vi "SyncTag_2.0 Test.vi"() -> ()   [LabVIEW 2017]
uses:
  <vilib>/Utility/error.llb/DialogType.ctl
  <vilib>/DAQmx/write.llb/DAQmx Write (Digital Wfm 1Chan NSamp).vi
  <vilib>/Waveform/DWDTOps.llb/DWDT Digital Size.vi
  <vilib>/DAQmx/create/channels.llb/DAQmx Create Channel (CO-Pulse Generation-Time).vi
  <vilib>/DAQmx/configure/timing.llb/DAQmx Timing (Implicit).vi
  <vilib>/DAQmx/create/channels.llb/DAQmx Create Channel (DO-Digital Output).vi
  <vilib>/DAQmx/configure/timing.llb/DAQmx Timing (Sample Clock).vi
  <vilib>/Waveform/DWDTOps.llb/DWDT Boolean Array to Digital.vi
  <vilib>/Waveform/DWDTOps.llb/DWDT Uncompress Digital.vi
  <vilib>/DAQmx/miscellaneous.llb/DAQmx Fill In Error Info.vi
panel:
  out "error out 8":errorcluster
  out "error out 7":errorcluster
  out "Numeric":i32
  out "error out 6":errorcluster
  out "error out 5":errorcluster
  out "error out 4":errorcluster
  out "error out 3":errorcluster
  out "error out 2":errorcluster
  out "error out":errorcluster
  in  "Sync Tagging":T1(tab)
  out "Minimum tagging period (pws)":u32=87
  out "Total tag data length (pws)":u32=86
  in  "TaggingPeriod (pws)":u32=155
  out "Tag data does NOT fit in period!!!":bool
  in  "Calculate recommended tag settings":bool
  in  "Validate tag settings":bool
  in  "TagMarkerDuration (pws)":i32=10
  in  "stop":bool
  out "Digital Waveform Graph":digitalwaveform(graph)
  in  "Minimum extra tag separation (pws)":u32=1
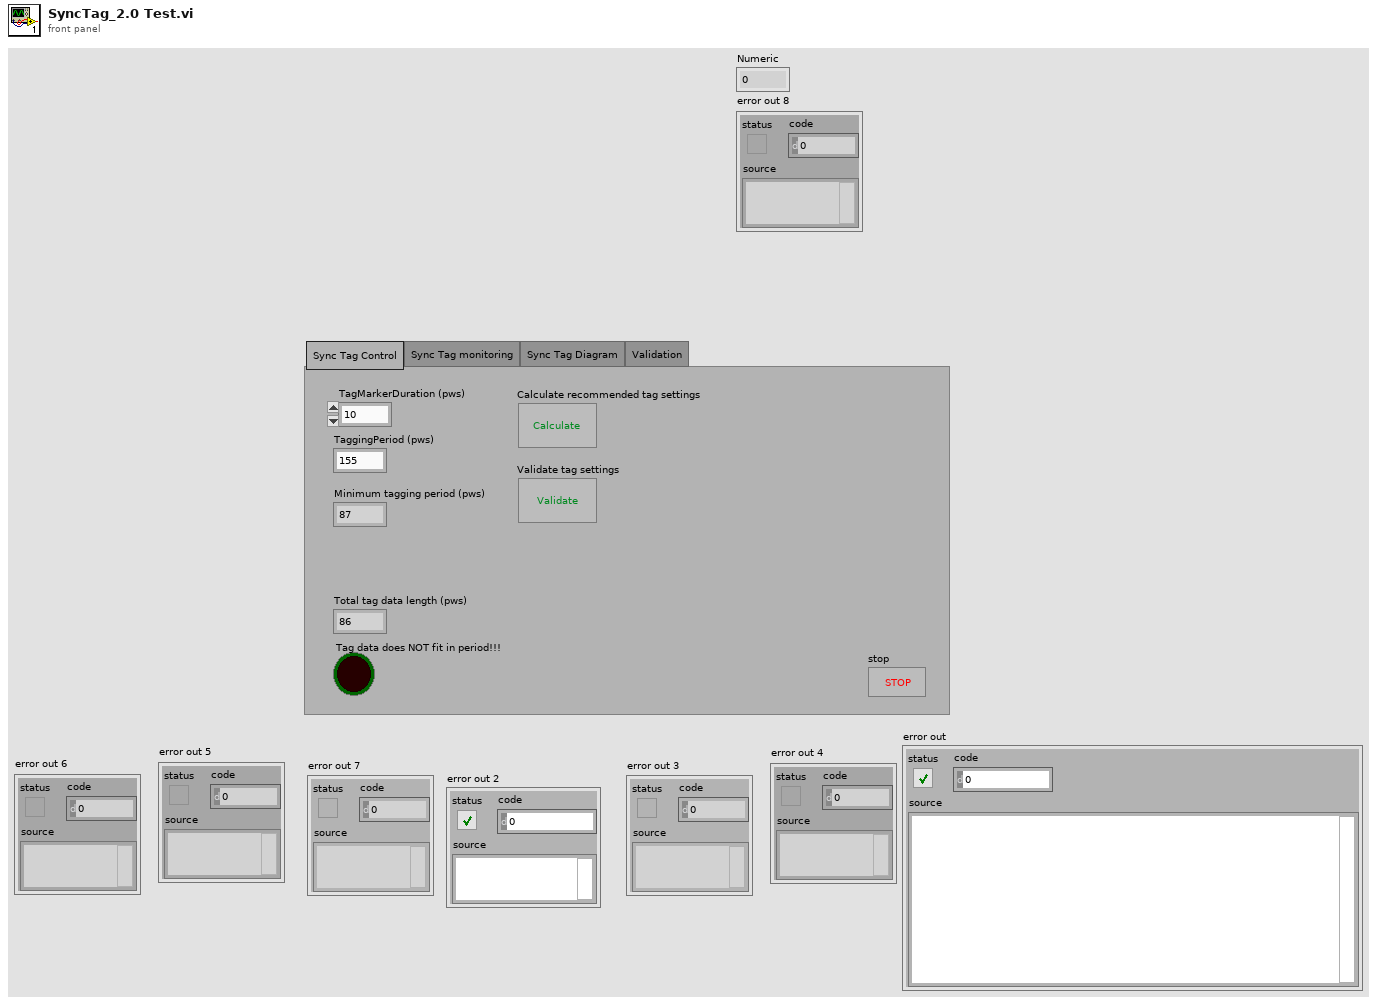
[diagram p1: front panel]
types:
  T1 = enum32{"Sync Tag Control", "Sync Tag monitoring", "Sync Tag Diagram", "Validation"}
  T2 = typedef "DialogType.ctl" = u16
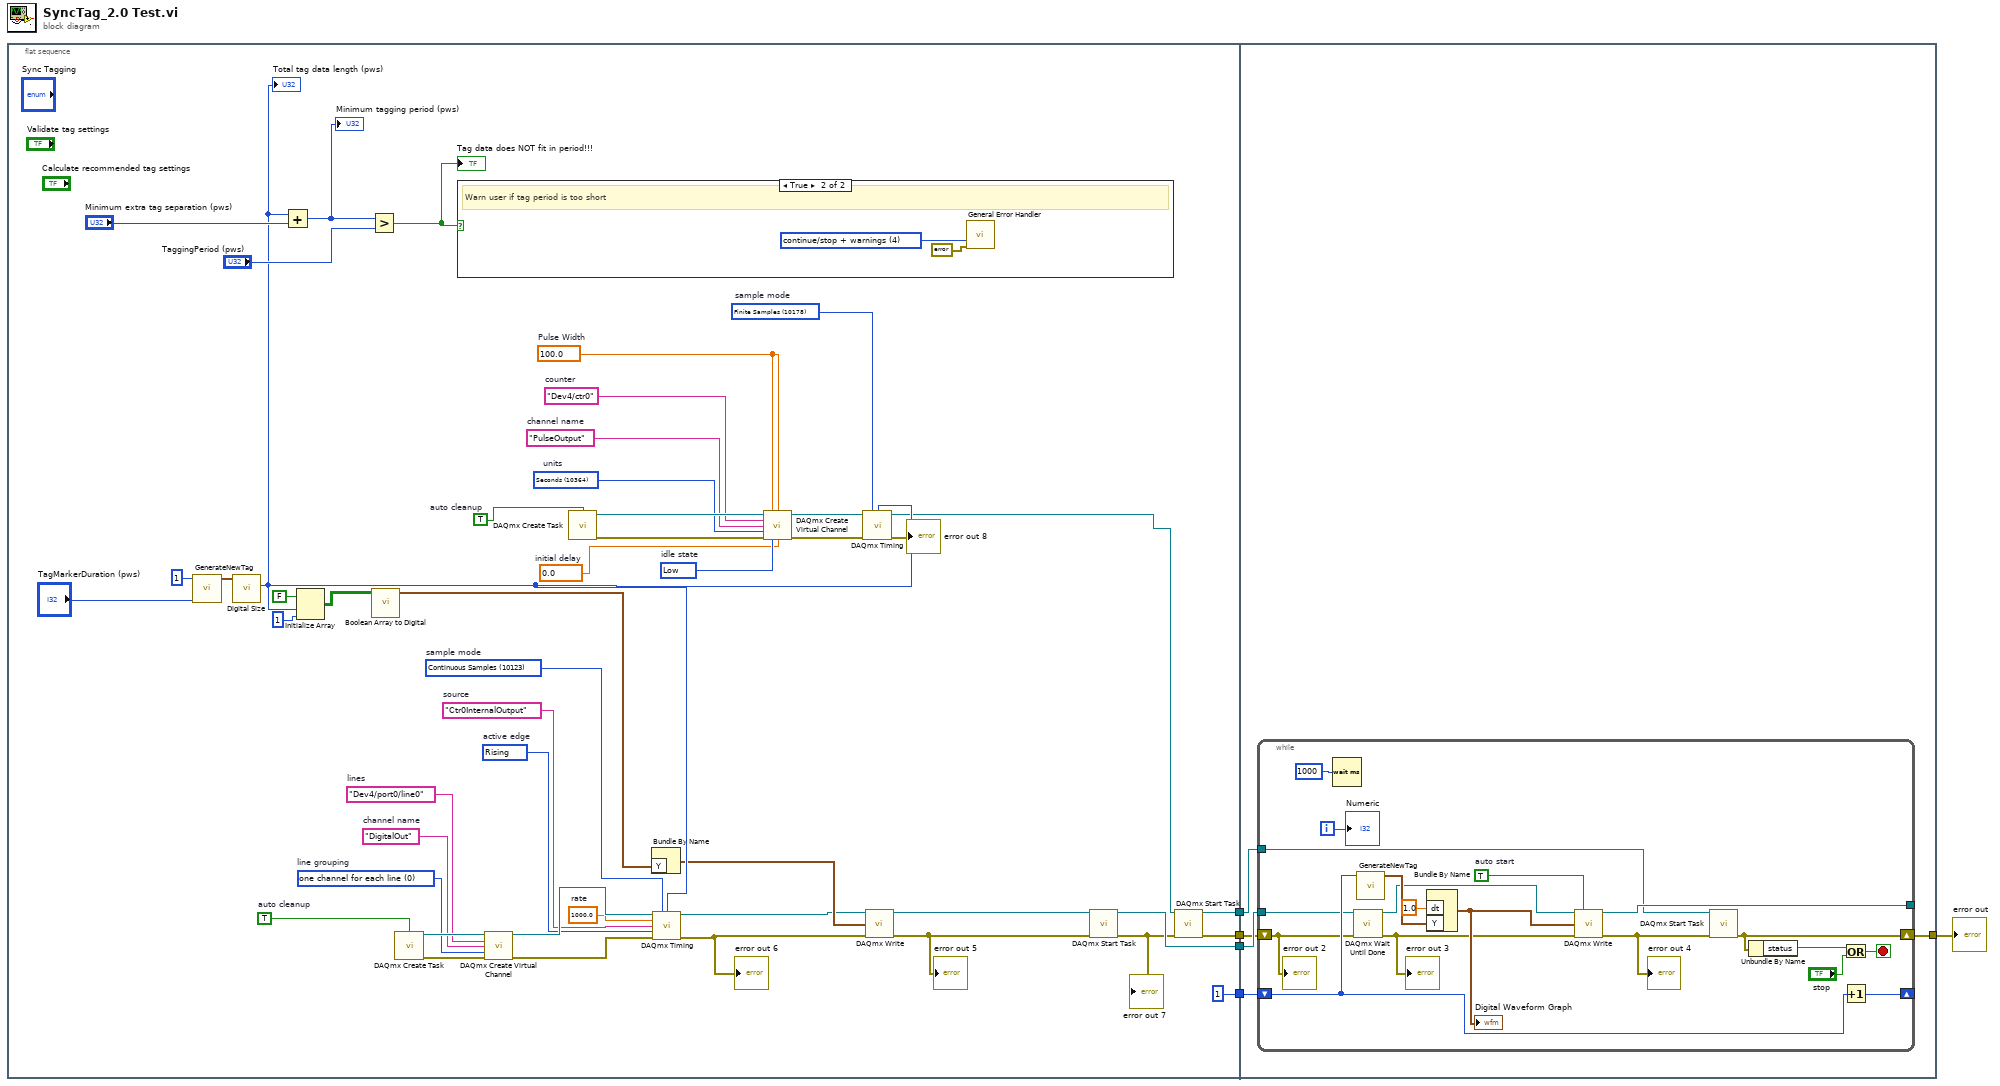
[diagram p0: block diagram]
diagram:
  n1 = flat-sequence {
    tunnel: [w8] -> w5
    tunnel: [u32 1 ("Tag num")] -> w4
    tunnel: [w13] -> w3
    tunnel: [w9] -> w1
    tunnel: w5 -> [w60]
    tunnel: w4 -> [w59]
    tunnel: w3 -> [w58]
    tunnel: [w57] -> w2
    tunnel: w1 -> [w56]
    frame #0 {
      w30 = 10123 items=["Finite Samples"=10178, "Continuous Samples"=10123, "Hardware Timed Single Point"=12522]  # sample mode
      w29 = 1000.0  # rate
      w27 = 10280 items=["Rising"=10280, "Falling"=10171]  # active edge
      w28 = "Ctr0InternalOutput"  # source
      w24 = 0 items=["one channel for each line", "one channel for all lines"]  # line grouping
      w25 = "DigitalOut"  # channel name
      w26 = "Dev4/port0/line0"  # lines
      w23 = TRUE  # auto cleanup
      w22 = 10178 items=["Finite Samples"=10178, "Continuous Samples"=10123, "Hardware Timed Single Point"=12522]  # sample mode
      w21 = 100.0  # Pulse Width
      w16 = 0.0  # initial delay
      w17 = 10214 items=["High"=10192, "Low"=10214]  # idle state
      w18 = 10364 items=["Seconds"=10364, "From Custom Scale"=10065]  # units
      w19 = "PulseOutput"  # channel name
      w20 = "Dev4/ctr0"  # counter
      w15 = TRUE  # auto cleanup
      n2 = call "GenerateNewTag.vi"("TagMarkerDuration (pws)"="TagMarkerDuration (pws)", "Tag num"=u32 1) -> ("digital waveform"=w46:digitalwaveform)  [unwired: 9 in]
      n3 = call-poly <vilib>:"Digital Size.vi"("digital waveform in"=w46) -> ("number of samples"=w47:i32)  [unwired: 7 in, 3 out]
      "Total tag data length (pws)" <- w47
      n4 = Add(x=w47, y="Minimum extra tag separation (pws)") -> (x+y=w53:u32)
      "Minimum tagging period (pws)" <- w53
      n5 = Initialize Array(FALSE, w47, 1 ("dimension size")) -> (w43:bool[][])
      n6 = Greater?(x=w53, y="TaggingPeriod (pws)") -> (0:w52:bool)
      "Tag data does NOT fit in period!!!" <- w52
      n7 = call-poly <vilib>:"Boolean Array to Digital.vi"("boolean array"=w43) -> ("digital waveform"=w44:digitalwaveform)  [unwired: 9 in, 1 out]
      n8 = call <vilib>:"DAQmx Create Task.vi"("auto cleanup"=w23) -> ("task out"=w40:refnum<k21>, "error out"=w39:errorcluster)  [unwired: 13 in]
      n9 = case shown="True" w52 {
        frame False {
        }
        frame True {
          w54 = T2 4 items=["no dialog", "OK message", "continue or stop message", "OK message + warnings", "continue/stop + warnings"] ("type of dialog (OK msg:1)")
          # "Warn user if tag period is too short"
          n10 = call <vilib>:"General Error Handler.vi"("type of dialog (OK msg:1)"=w54, "error in (no error)"=errorcluster {"status"=TRUE, "code"=-1967345148, "source"="Warning! Tag data does not fit in period. \nPlease increase tag period and restart VI."}) -> ()  [unwired: 9 in, 5 out]
        }
      }
      n11 = call-poly <vilib>:"DAQmx Create Virtual Channel.vi"("task in"=w40, "lines"=w26, "name to assign"=w25, "line grouping"=w24, "error in"=w39) -> ("task out"=w42:refnum<k21>, "error out"=w41:errorcluster)  [unwired: 9 in]
      n12 = call <vilib>:"DAQmx Create Task.vi"("auto cleanup"=w15) -> ("task out"=w34:refnum<k21>, "error out"=w33:errorcluster)  [unwired: 13 in]
      n13 = Bundle By Name("Y"=w44) -> (w45:digitalwaveform)  [unwired: 1 in]
      n14 = call-poly <vilib>:"DAQmx Timing.vi"("task/channels in"=w42, "sample mode"=w30, "samples per channel"=w47, "rate"=w29, "source"=w28, "active edge"=w27, "error in"=w41) -> ("task out"=w11:refnum<k21>, "error out"=w12:errorcluster)  [unwired: 7 in]
      "error out 6" <- w12
      n15 = call-poly <vilib>:"DAQmx Create Virtual Channel.vi"("task in"=w34, "high time"=w21, "low time"=w21, "counter"=w20, "name to assign"=w19, "units"=w18, "error in"=w33, "idle state"=w17, "initial delay"=w16) -> ("task out"=w36:refnum<k21>, "error out"=w35:errorcluster)  [unwired: 5 in]
      n16 = call-poly <vilib>:"DAQmx Timing.vi"("task/channels in"=w36, "sample mode"=w22, "samples per channel"=w47, "error in"=w35) -> ("task out"=w7:refnum<k21>, "error out"=→"error out 8":errorcluster)  [unwired: 10 in]
      n17 = call-poly <vilib>:"DAQmx Write.vi"("task/channels in"=w11, "data"=w45, "error in"=w12) -> ("task out"=w37:refnum<k21>, "error out"=w38:errorcluster)  [unwired: 10 in, 1 out]
      "error out 5" <- w38
      n18 = call <vilib>:"DAQmx Start Task.vi"("task/channels in"=w37, "error in"=w38) -> ("task out"=w13:refnum<k21>, "error out"=w10:errorcluster)  [unwired: 12 in]
      "error out 7" <- w10
      n19 = call <vilib>:"DAQmx Start Task.vi"("task/channels in"=w7, "error in"=w10) -> ("task out"=w8:refnum<k21>, "error out"=w9:errorcluster)  [unwired: 12 in]
    }
    frame #1 {
      n20 = while "Check for errors or stop pressed" {
        tunnel: [w76] -> _
        shift-right: [w68] -> w57
        shift-left: w56 -> [w63]
        tunnel: w60 -> [w70]
        shift-right: [w66] -> _
        shift-left: w59 -> [w67]
        tunnel: w58 -> [w65]
        i -> [w61]
        stop <- w78 stop-if-true
        w74 = TRUE  # auto start
        n21 = Wait (ms)(milliseconds to wait=u32 1000) -> ()  [unwired: 1 out]
        n22 = call <vilib>:"DAQmx Wait Until Done.vi"("task/channels in"=w65, "error in"=w63) -> ("task out"=w64:refnum<k21>, "error out"=w62:errorcluster)  [unwired: 12 in]
        "error out 3" <- w62
        n23 = call "GenerateNewTag.vi"("Tag num"=w67) -> ("digital waveform"=w73:digitalwaveform)  [unwired: 10 in]
        n24 = Bundle By Name("dt"=1.0, "Y"=w73) -> (w71:digitalwaveform)  [unwired: 1 in]
        "Digital Waveform Graph" <- w71
        n25 = call-poly <vilib>:"DAQmx Write.vi"("task/channels in"=w64, "auto start"=w74, "data"=w71, "error in"=w62) -> ("task out"=w76:refnum<k21>, "error out"=w69:errorcluster)  [unwired: 9 in, 1 out]
        "error out 4" <- w69
        n26 = call <vilib>:"DAQmx Start Task.vi"("task/channels in"=w70, "error in"=w69) -> ("error out"=w68:errorcluster)  [unwired: 12 in, 1 out]
        n27 = Unbundle By Name(w68) -> ("status"=w75:bool)
        n28 = Or(x=w75, y="stop") -> (x .or. y?=w78:bool)
        n29 = Increment(x=w67) -> (x+1=w66:u32)
        "error out 2" <- w63
        "Numeric" <- w61
      }
    }
  }
  "error out" <- w2
